vi "determine valubility.vi"() -> ()   [LabVIEW 2009]
uses:
  <vilib>/Utility/file.llb/Write To Spreadsheet File (I64).vi
  <vilib>/Analysis/NI_AALBase.lvlib
panel:
  in  "intervals":i32=25
  out "Histogram Graph":T1(graph)
  out "bar graph":cluster{i32[], dbl[]}[](graph)
  in  "median":dbl=16.0
  in  "Abort":bool
  in  "folders":cluster{"file path":path, "depth":i32}[](array[cluster])
  out "mini progress":i32(slide) scale=-1.1..1255.0
  in  "seeding data":T2={"read seed value from file"=FALSE, "seed source file path"=path "", "indexes"={"index"=2, "index 2"=3}, "subtract from"=0.0}
  in  "result ordering":enum32{"by ranking", "by number"}(radio)=enum."by number"
  in  "save results?":bool
  out "main progress":i32(slide) scale=-1.1..9.0
  out "results":T3(array[cluster])
  in  "iterations":i32=10
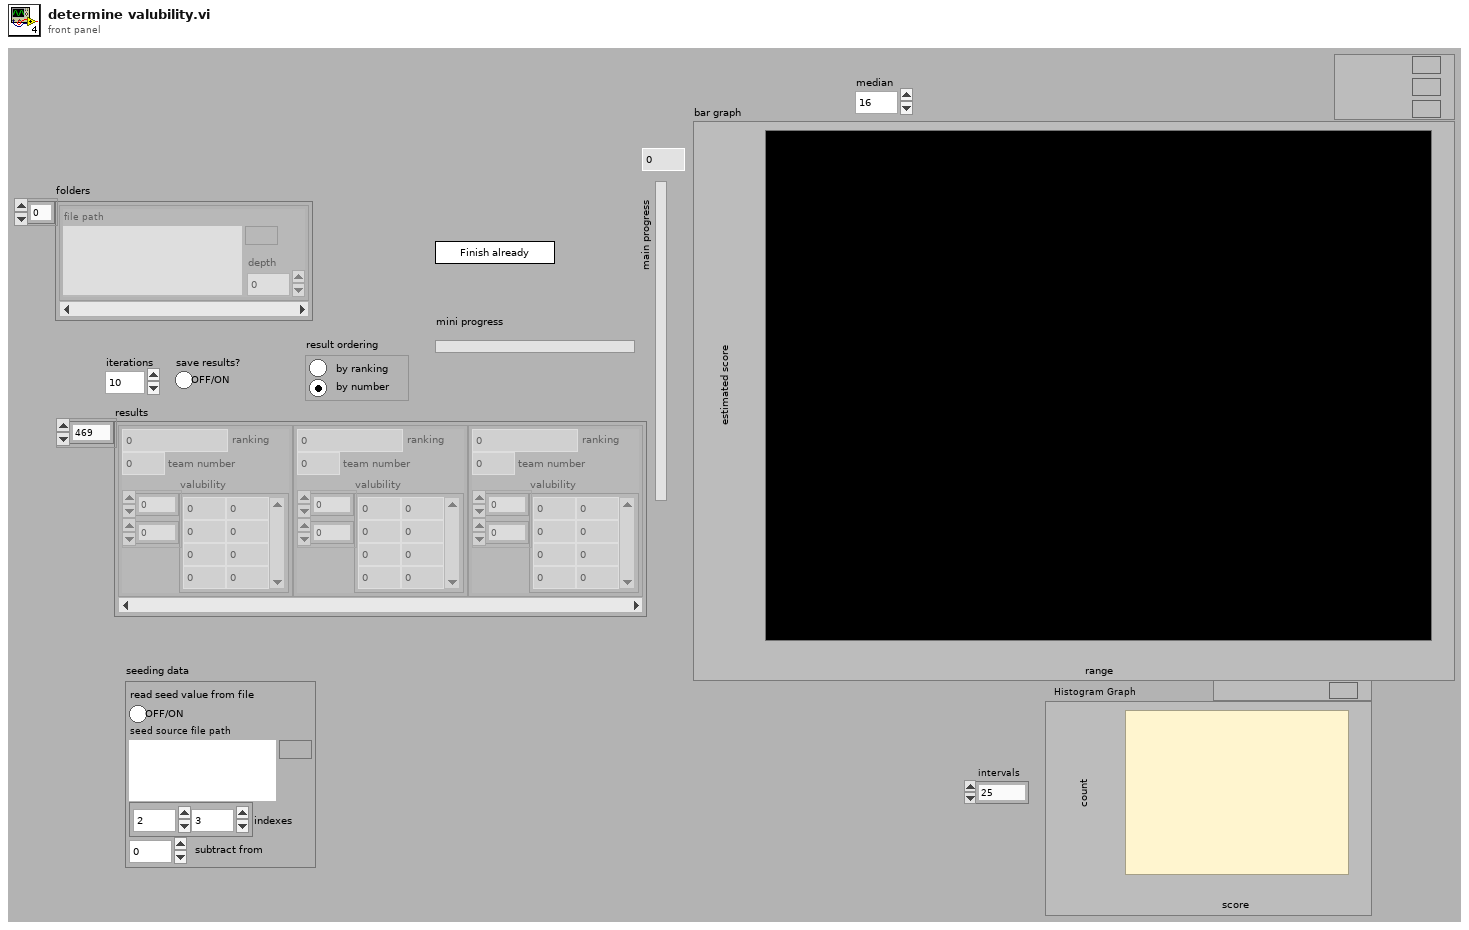
[diagram p1: front panel]
types:
  T1 = cluster{"X Values":dbl[], "Histogram: h(x)":i32[]}
  T2 = cluster{"read seed value from file":bool, "seed source file path":path, "indexes":cluster{"index":i32, "index 2":i32}, "subtract from":dbl}
  T3 = cluster{"ranking":dbl, i16, "valubility":dbl[][]}[]
  T4 = cluster{i16, "scores":i16[][], "valubility":dbl[][]}[]
  T5 = cluster{i16, "scores":i16[][], "valubility":dbl[][]}
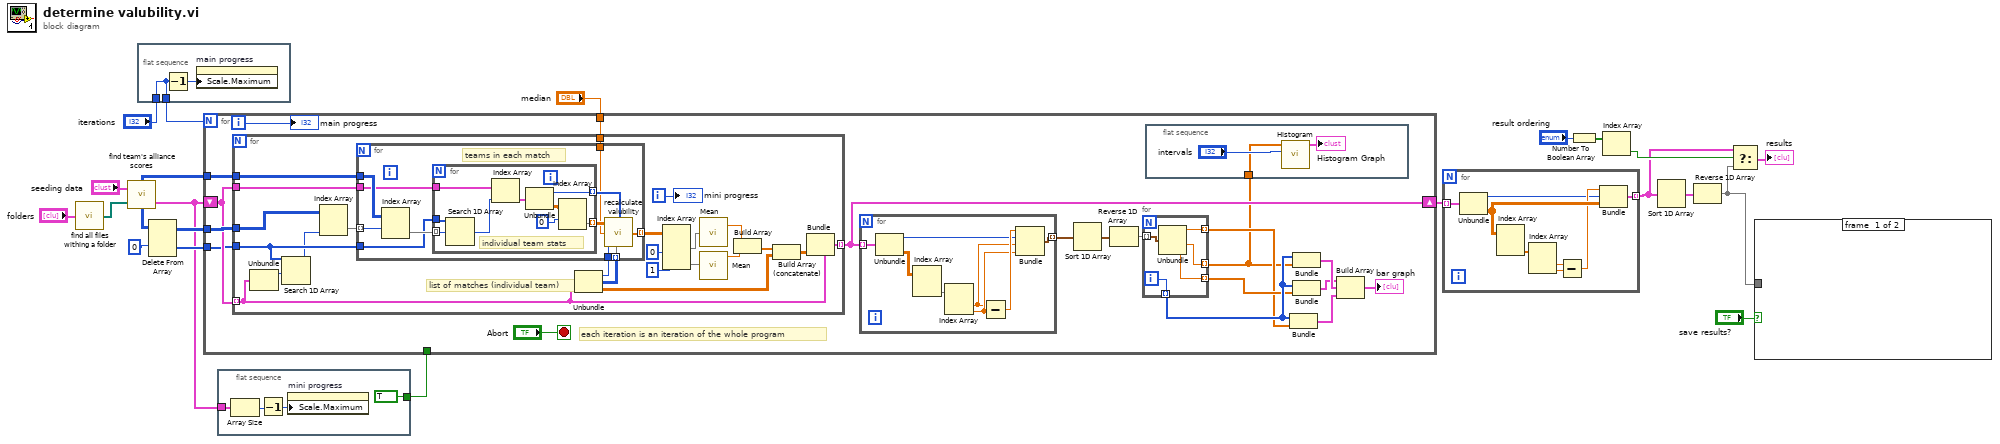
[diagram p0: block diagram]
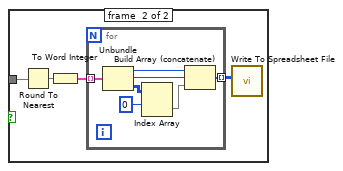
[diagram p2: hidden frame]
diagram:
  n1 = call "find all files withing a folder.vi"("folders"="folders") -> ("paths"=w3:path[])  [unwired: 1 out]
  n2 = call "find team's alliance scores.vi"("Data sources"=w3, "seeding data"="seeding data") -> ("team/match locator"=w21:i16[][], "Array"=w5:T4, "alliance info"=w22:i16[][])  [unwired: 1 out]
  n3 = flat-sequence {
    tunnel: "iterations" -> [w23]
    tunnel: [w23] -> w15
    frame #0 {
      n4 = Decrement(x=w23) -> (x-1=w24:i32)
      n5 = property on="main progress" class="Slide (strict)"("Scale.Maximum"=w24) -> ()  [unwired: 2 in, 2 out]
    }
  }
  n6 = Delete From Array(array=w21, index (row)=0) -> (deleted portion=w18:i16[], array with subset deleted=w20:i16[][])  [unwired: 2 in]
  n7 = for {
    N: w15 -> [_]
    shift-right: [w28] -> w19
    shift-left: w5 -> [w41]
    tunnel: w20 -> [w43]
    tunnel: w22 -> [w42]
    tunnel: w18 -> [w40]
    tunnel: w4 -> [_]
    tunnel: "median" -> [w34]
    i -> [w39]
    stop <- "Abort" stop-if-true
    # "each iteration is an iteration of the whole program"
    n8 = for {
      tunnel: w41 -> [w80]
      tunnel: w43 -> [w64]
      tunnel: w42 -> [w81]
      tunnel: [w68] -> w28 mode=indexing
      tunnel: w41 -> [w66] mode=indexing
      tunnel: w40 -> [w67]
      tunnel: w34 -> [w60]
      i -> [w61]
      # "list of matches (individual team)"
      n9 = Unbundle(w66) -> (w65:i16)  [unwired: 2 out]
      n10 = Search 1D Array(1D array=w67, element=w65) -> (index of element=w62:i32)  [unwired: 1 in]
      n11 = Index Array(array=w64, index (col)=w62) -> (element=w63:i16[])  [unwired: 1 in]
      n12 = Unbundle(w66) -> (w79:i16, "scores"=w82:i16[][], "valubility"=w70:dbl[][])
      n13 = for {
        tunnel: w82 -> [w87] mode=indexing
        tunnel: w80 -> [w92]
        tunnel: w81 -> [w93]
        tunnel: w63 -> [w84] mode=indexing
        tunnel: w79 -> [w90]
        tunnel: [w86] -> w78 mode=indexing
        tunnel: w67 -> [w85]
        tunnel: w60 -> [w83]
        # "teams in each match"
        n14 = Index Array(array=w93, index (row)=w84) -> (element=w91:i16[])  [unwired: 1 in]
        n15 = for {
          tunnel: w91 -> [w96] mode=indexing
          tunnel: w92 -> [w102]
          tunnel: [w98] -> w88 mode=indexing
          tunnel: [w97] -> w89 mode=indexing
          tunnel: w85 -> [w95]
          # "individual team stats"
          n16 = Search 1D Array(1D array=w95, element=w96) -> (index of element=w94:i32)  [unwired: 1 in]
          n17 = Index Array(array=w102, index=w94) -> (element=w101:T5)
          n18 = Unbundle(w101) -> (w97:i16, "valubility"=w100:dbl[][])  [unwired: 1 out]
          n19 = Index Array(array=w100, index (row)=0) -> (element=w98:dbl[])  [unwired: 1 in]
        }
        n20 = call "recalculate valubility.vi"("valubility"=w88, "teams in match"=w89, "median"=w83, "team number"=w90, "scores"=w87) -> ("valubility"=w86:dbl[])  [unwired: 3 in, 1 out]
      }
      n21 = Index Array(array=w78, index (col) #1=0 ("disabled index (col)"), index (col) #2=1 ("index (col)")) -> (element #1=w75:dbl[], element #2=w74:dbl[])  [unwired: 2 in]
      n22 = call <vilib>:"Mean.vi"("X"=w75) -> ("mean"=w73:dbl)  [unwired: 1 out]
      n23 = call <vilib>:"Mean.vi"("X"=w74) -> ("mean"=w72:dbl)  [unwired: 1 out]
      n24 = Build Array(w73, w72) -> (w71:dbl[])
      n25 = Build Array (concatenate)(w71, w70) -> (w69:dbl[][])
      n26 = Bundle(cluster=w66, "valubility"=w69) -> (w68:T5)  [unwired: 2 in]
      "mini progress" <- w61
    }
    n27 = for {
      tunnel: w28 -> [w54] mode=indexing
      tunnel: [w52] -> w29 mode=indexing
      n28 = Unbundle(w54) -> (w49:i16, "valubility"=w51:dbl[][])  [unwired: 1 out]
      n29 = Index Array(array=w51) -> (element=w53:dbl[])  [unwired: 2 in]
      n30 = Index Array(array=w53) -> (element #1=w47:dbl, element #2=w48:dbl)  [unwired: 2 in]
      n31 = Subtract(x=w47, y=w48) -> (x-y=w50:dbl)
      n32 = Bundle(w50, w49, "value"=w47, "value"=w48) -> (w52:cluster{dbl, i16, "value":dbl, "value":dbl})  [unwired: 1 in]
    }
    n33 = Sort 1D Array(array=w29) -> (sorted array=w30:cluster{dbl, i16, "value":dbl, "value":dbl}[])
    n34 = Reverse 1D Array(array=w30) -> (reversed array=w27:cluster{dbl, i16, "value":dbl, "value":dbl}[])
    n35 = for {
      tunnel: w27 -> [w59] mode=indexing
      tunnel: [w56] -> w25 mode=indexing
      tunnel: [w55] -> w32 mode=indexing
      tunnel: [w58] -> w33 mode=indexing
      tunnel: [w57] -> w26 mode=indexing
      i -> [w58]
      n36 = Unbundle(w59) -> (w57:dbl, "value"=w56:dbl, "value"=w55:dbl)  [unwired: 1 out]
    }
    n37 = flat-sequence {
      tunnel: w25 -> [w44]
      frame #0 {
        n38 = call <vilib>:"Histogram.vi"("intervals"="intervals", "X"=w44) -> ("Histogram Graph"=→"Histogram Graph":T1)  [unwired: 6 in, 3 out]
      }
    }
    n39 = Bundle(w33, w26) -> (w31:cluster{i32[], dbl[]})  [unwired: 1 in]
    n40 = Bundle(w33, w25) -> (w36:cluster{i32[], dbl[]})  [unwired: 1 in]
    n41 = Bundle(w33, w32) -> (w35:cluster{i32[], dbl[]})  [unwired: 1 in]
    n42 = Build Array(w35, w36, w31) -> (→"bar graph":cluster{i32[], dbl[]}[])
    "main progress" <- w39
  }
  n43 = flat-sequence {
    tunnel: w5 -> [w106]
    tunnel: [TRUE] -> w4
    frame #0 {
      n44 = Array Size(array=w106) -> (size(s)=w105:i32)
      n45 = Decrement(x=w105) -> (x-1=w104:i32)
      n46 = property on="mini progress" class="Slide (strict)"("Scale.Maximum"=w104) -> ()  [unwired: 2 in, 2 out]
    }
  }
  n47 = for {
    tunnel: w19 -> [w114] mode=indexing
    tunnel: [w110] -> w6 mode=indexing
    n48 = Unbundle(w114) -> (w107:i16, "valubility"=w109:dbl[][])  [unwired: 1 out]
    n49 = Index Array(array=w109) -> (element=w113:dbl[])  [unwired: 2 in]
    n50 = Index Array(array=w113) -> (element #1=w111:dbl, element #2=w112:dbl)  [unwired: 2 in]
    n51 = Subtract(x=w111, y=w112) -> (x-y=w108:dbl)
    n52 = Bundle(w108, w107, "valubility"=w109) -> (w110:cluster{dbl, i16, "valubility":dbl[][]})  [unwired: 1 in]
  }
  n53 = Number To Boolean Array(number="result ordering") -> (Boolean array=w11:bool[])
  n54 = Index Array(array=w11) -> (element=w10:bool)  [unwired: 1 in]
  n55 = Sort 1D Array(array=w6) -> (sorted array=w13:cluster{dbl, i16, "valubility":dbl[][]}[])
  n56 = Reverse 1D Array(array=w13) -> (reversed array=w7:cluster{dbl, i16, "valubility":dbl[][]}[])
  n57 = Select(t=w6, s=w10, f=w7) -> (s? t:f=→"results":cluster{dbl, i16, "valubility":dbl[][]}[])
  n58 = case shown="True" "save results?" {
    tunnel: w7 -> [_ w116]
    frame #0 {
    }
    frame #1 {
      n59 = Round To Nearest(number=w116) -> (nearest integer value=w117:cluster{dbl, i16, "valubility":dbl[][]}[])
      n60 = To Word Integer(number=w117) -> (16bit integer=w115:cluster{i16, i16, "valubility":i16[][]}[])
      n61 = for {
        tunnel: w115 -> [w125] mode=indexing
        tunnel: [w119] -> w118 mode=indexing
        n62 = Unbundle(w125) -> (w124:i16, w123:i16, "valubility"=w122:i16[][])
        n63 = Index Array(array=w122, index (row)=0) -> (element=w120:i16[])  [unwired: 1 in]
        n64 = Build Array (concatenate)(w124, w123, w120) -> (w119:i16[])
      }
      n65 = call-poly <vilib>:"Write To Spreadsheet File.vi"("2D data"=w118) -> ()  [unwired: 7 in, 1 out]
    }
  }
